vi "USB Close.vi"(8 "error in (no error)":errorcluster) -> (0 "error out":errorcluster, 3 "function return":i32)   [LabVIEW 2013, in "TimeTagLV.lvlib"]
doc: "LIBRARY_API int USB_Close();"
uses:
  TimeTagLV.lvlib
  TimeTag.dll
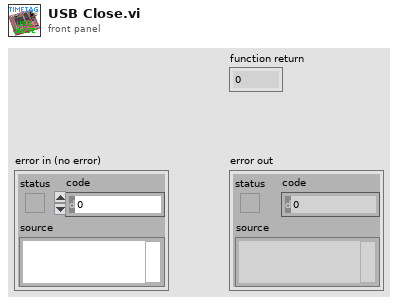
[diagram p1: front panel]
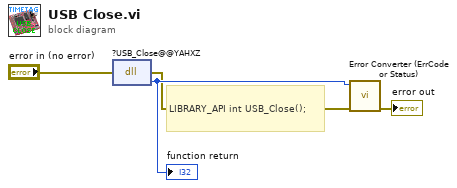
[diagram p0: block diagram]
diagram:
  # "LIBRARY_API int USB_Close();"
  n1 = dll-call lib="C:/FPGA_XyloEM/TimeTagDLL/TimeTagLV/TimeTag.*" fn="?USB_Close@@YAHXZ"(error in="error in (no error)") -> (error out=w2:errorcluster, w4:i32)  [unwired: 2 in, 1 out]
  "function return" <- w4
  n2 = call "Error Converter (ErrCode or Status).vi"("error in (no error)"=w2, "error code"=w4) -> ("error out"=→"error out":errorcluster)  [unwired: 9 in]
